vi "UDP test incomplete packet error.vi"() -> ()   [LabVIEW 2013, in "TEC tests.lvlib"]
uses:
  testing/TEC tests.lvlib
  <vilib>/NI/Tag Bus/table/data table.ctl
  <vilib>/NI/Tag Bus/table/data table.lvlib
panel:
  out "error out 4":errorcluster
  out "Numeric":i32
  in  "port2":u16=5556
  in  "port1":u16=5555
  out "error out 3":errorcluster
  out "error out 2":errorcluster
  out "error out":errorcluster
  in  "timeout ms (25000)":i32=1000
  in  "max size (548)":i32
  out "rx":string
  out "sent":string
  in  "stop 2":bool
  in  "read":bool
  in  "count to send":i32
  in  "send":bool
  in  "stop":bool
  # "windows drops whole packet if we don't read enough\nlinux rt drops remainder of packet"
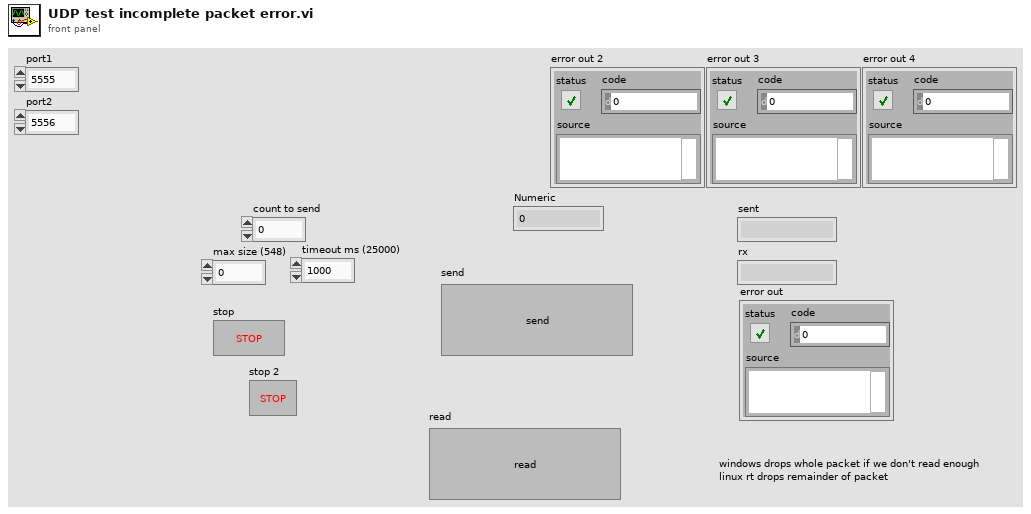
[diagram p1: front panel]
types:
  T1 = typedef "tag bus.lvlib/data table.lvlib/data table.ctl" = cluster{"Double":dbl[], "Single":sgl[], "I64":i64[], "I32":i32[], "I16":i16[], "I8":i8[], "U64":u64[], "U32":u32[], "U16":u16[], "U8":u8[], "Boolean":bool[], "String":string[], "Array of Double":cluster{"DBL Array":dbl[]}[], "Array of Single":cluster{"SGL Array":sgl[]}[], "Array of I64":cluster{"I64 Array":i64[]}[], "Array of I32":cluster{"I32 Array":i32[]}[], "Array of I16":cluster{"I16 Array":i16[]}[], "Array of I8":cluster{"I8 Array":i8[]}[], "Array of U64":cluster{"U64 Array":u64[]}[], "Array of U32":cluster{"U32 Array":u32[]}[], "Array of U16":cluster{"U16 Array":u16[]}[], "Array of U8":cluster{"U8 Array":u8[]}[], "Array of Boolean":cluster{"Boolean Array":bool[]}[], "Array of String":cluster{"String Array":string[]}[]}
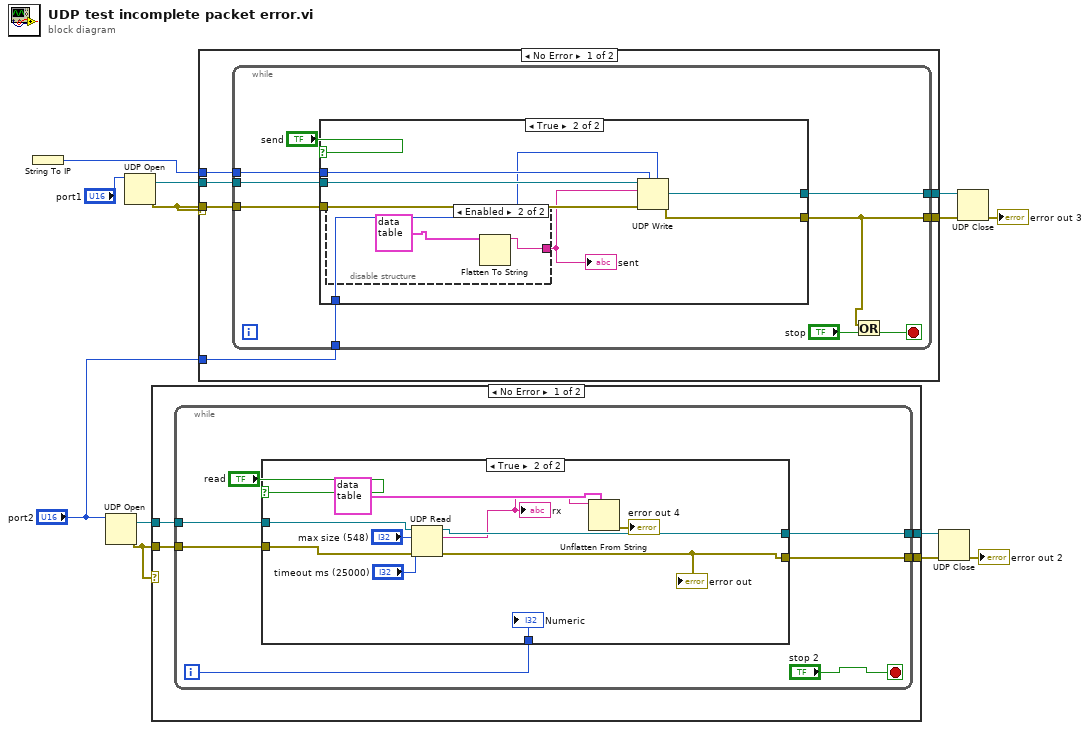
[diagram p0: block diagram]
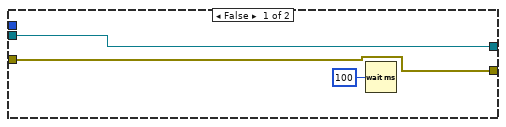
[diagram p2: hidden frame]
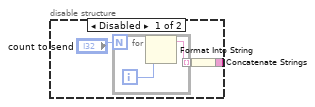
[diagram p3: hidden frame]
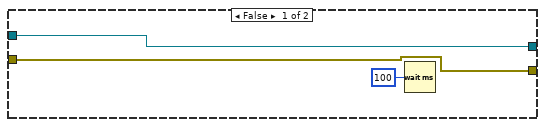
[diagram p5: hidden frame]
diagram:
  n1 = String To IP() -> (0:w9:u32)  [unwired: 1 in]
  n2 = UDP Open(11:"port2") -> (port=w6:refnum<k16>, 0:w5:errorcluster)  [unwired: 4 in, 1 out]
  n3 = UDP Open(11:"port1") -> (port=w13:refnum<k16>, 0:w2:errorcluster)  [unwired: 4 in, 1 out]
  n4 = case shown="No Error" w5 {
    tunnel: [w17 w39] -> w8
    tunnel: [w16 w38] -> w7
    tunnel: w5 -> [w15 w39]
    tunnel: w6 -> [w14 w38]
    frame No Error {
      n5 = while {
        tunnel: w14 -> [w23]
        tunnel: w15 -> [w22]
        tunnel: [w21] -> w16
        tunnel: [w20] -> w17
        i -> [w18]
        stop <- "stop 2" stop-if-true
        n6 = case shown="True" "read" {
          tunnel: w23 -> [w26 w37]
          tunnel: w22 -> [w25 w36]
          tunnel: [w26 w35] -> w21
          tunnel: [w25 w34] -> w20
          tunnel: w18 -> [_ w31]
          frame False {
            n7 = Wait (ms)(milliseconds to wait=u32 100) -> ()  [unwired: 1 out]
          }
          frame True {
            n8 = UDP Read(connection ID=w37, max size (548)="max size (548)", timeout ms (25000)="timeout ms (25000)", 8:w36) -> (data out=w29:string, error out=w34:errorcluster, 3:w35:refnum<k16>)  [unwired: 2 out]
            "rx" <- w29
            "error out" <- w34
            n9 = Unflatten From String(type=T1 {"Double"=[], "Single"=[], "I64"=[], "I32"=[], "I16"=[], "I8"=[], "U64"=[], "U32"=[], "U16"=[], "U8"=[], "Boolean"=[], "String"=[], "Array of Double"=[], "Array of Single"=[], "Array of I64"=[], "Array of I32"=[], "Array of I16"=[], "Array of I8"=[], "Array of U64"=[], "Array of U32"=[], "Array of U16"=[], "Array of U8"=[], "Array of Boolean"=[], "Array of String"=[]} ("data table"), binary string=w29) -> (error out=→"error out 4":errorcluster)  [unwired: 3 in, 2 out]
            "Numeric" <- w31
          }
        }
      }
    }
    frame Error {
    }
  }
  n10 = case shown="No Error" w2 {
    selector: w2 -> [_ w72]
    tunnel: w13 -> [w45 w73]
    tunnel: w2 -> [w44 _]
    tunnel: [w43 w73] -> w12
    tunnel: [w42 w72] -> w11
    tunnel: w9 -> [w41 _]
    tunnel: "port2" -> [w40 _]
    frame No Error {
      n11 = while {
        tunnel: w45 -> [w52]
        tunnel: w44 -> [w51]
        tunnel: [w50] -> w43
        tunnel: [w47] -> w42
        tunnel: w41 -> [w49]
        tunnel: w40 -> [w46]
        stop <- w48 stop-if-true
        n12 = case shown="True" "send" {
          tunnel: w52 -> [w56 w64]
          tunnel: w51 -> [w55 w63]
          tunnel: [w56 w62] -> w50
          tunnel: [w55 w61] -> w47
          tunnel: w49 -> [_ w60]
          tunnel: w46 -> [_ w59]
          frame False {
            n13 = Wait (ms)(milliseconds to wait=u32 100) -> ()  [unwired: 1 out]
          }
          frame True {
            n14 = disable-structure shown="Enabled" {
              disable-tunnel: [w65 w71] -> w58
              frame Disabled {
                n15 = for {
                  N: "count to send" -> [_]
                  tunnel: [w68] -> w66 mode=indexing
                  i -> [w69]
                  n16 = Format Into String(w69) -> (resulting string=w68:string)  [unwired: 3 in, 1 out]
                }
                n17 = Concatenate Strings(w66) -> (w65:string)
              }
              frame Enabled {
                n18 = Flatten To String(anything=T1 {"Double"=[0.0, 0.0, 0.0, 0.0, 0.0, 0.0, 0.0, 0.0, 0.0, 0.0, 0.0, 0.0, 0.0, 0.0, 0.0, 0.0, 0.0, 0.0, 0.0, 0.0, 0.0, 0.0, 0.0, 0.0, 0.0, 0.0, 0.0, 0.0, 0.0, 0.0, 0.0, 0.0, 0.0, 0.0, 0.0, 0.0, 0.0, 0.0, 0.0, 0.0, 0.0, 0.0, 0.0, 0.0, 0.0, 0.0, 0.0, 0.0, 0.0, 0.0, 0.0, 0.0, 0.0, 0.0, 0.0, 1.0], "Single"=[0.0, 0.0, 0.0, 0.0, 0.0, 0.0, 0.0, 0.0, 0.0, 0.0, 0.0, 0.0, 0.0, 0.0, 0.0, 0.0, 0.0, 0.0, 0.0, 0.0, 0.0, 0.0, 0.0, 0.0, 0.0, 0.0, 0.0, 0.0, 0.0, 0.0, 0.0, 0.0, 0.0, 1.0], "I64"=[2], "I32"=[], "I16"=[], "I8"=[], "U64"=[], "U32"=[], "U16"=[], "U8"=[], "Boolean"=[], "String"=[], "Array of Double"=[{"DBL Array"=[]}, {"DBL Array"=[1.0]}], "Array of Single"=[], "Array of I64"=[], "Array of I32"=[], "Array of I16"=[], "Array of I8"=[], "Array of U64"=[], "Array of U32"=[], "Array of U16"=[], "Array of U8"=[], "Array of Boolean"=[], "Array of String"=[]} ("data table in")) -> (data string=w71:string)  [unwired: 3 in, 2 out]
              }
            }
            "sent" <- w58
            n19 = UDP Write(address=w60, port or service name=w59, connection ID=w64, data in=w58, 8:w63) -> (error out=w61:errorcluster, 3:w62:refnum<k16>)  [unwired: 1 in]
          }
        }
        n20 = Or(x=w47, y="stop") -> (x .or. y?=w48:bool)
      }
    }
    frame Error {
    }
  }
  n21 = UDP Close(connection ID=w7, 8:w8) -> (error out=→"error out 2":errorcluster)  [unwired: 1 out]
  n22 = UDP Close(connection ID=w12, 8:w11) -> (error out=→"error out 3":errorcluster)  [unwired: 1 out]
